vi "main.vi"() -> ()   [LabVIEW 2012]
panel:
  in  "请输入你需要的网址：":string="http://127.0.0.1/index.html"
  in  "Google Earth部分":refnum<k7>(container)
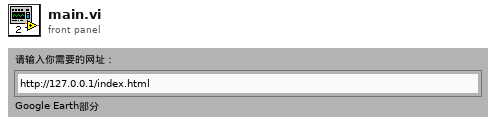
[diagram p1: front panel]
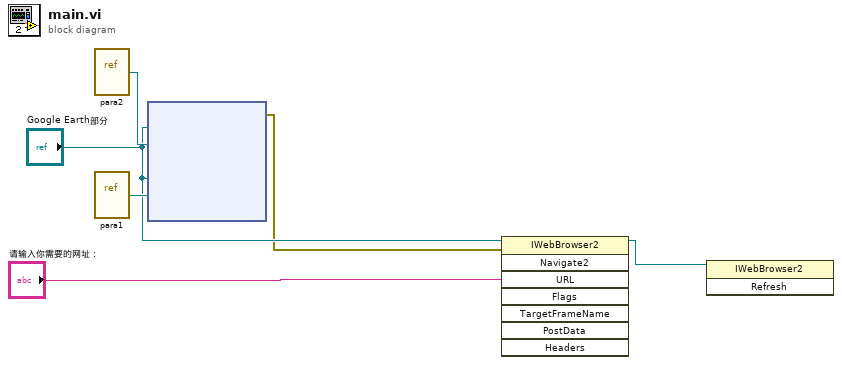
[diagram p0: block diagram]
diagram:
  n1 = vi-ref "para2.vi"() -> ("vi reference"=w6:refnum<vi>)
  n2 = vi-ref "para1.vi"() -> ("vi reference"=w5:refnum<vi>)
  n3 = node("Google Earth部分", w6, "Google Earth部分", w5) -> (w2:errorcluster)  [unwired: 4 in, 1 out]
  n4 = invoke class="IWebBrowser2" method="Navigate2"(reference="Google Earth部分", error in=w2, "URL"="请输入你需要的网址：") -> (reference out=w1:refnum<k7>)  [unwired: 5 in, 7 out]
  n5 = invoke class="IWebBrowser2" method="Refresh"(reference=w1) -> ()  [unwired: 2 in, 3 out]
